vi "MI Sync with Triggering (MAIN) repeatability.vi"(10 "FGENs":refnum<k15>[](array[refnum])=["FGEN1", "FGEN2"] caption="Resource Name", 11 "Scopes":refnum<k15>[](array[refnum])=["SCOPE1", "SCOPE2"] caption="resource name") -> (2 "Waveform Graph":waveform(dbl)[](graph), 3 "relative trigger position (s)":dbl[](array[numeric]) format="%#.3p")   [LabVIEW 2024]
doc: "This VI is a one shot example of synchronising 2x arb with 2 and 1 channels with 2x scopes with 2 and 1 channel.\nThe frequency the arb are to produce is set on the front panel and all are identical amplitude and frequency with the phase set to a 120 degree difference.\nTriggering of the oscilloscope is based on channel 0 of the first specified scope module as the signal crosses zero.\nWIthout using TCLK, triggering happens by preparing the FGEN first and starting their output when the master SCOPE which is set to reference trigger on ch0 passes out it's ready for start event. The second scope uses the reference trigger event from the first scope to start."
uses:
  <instrlib>/niScope/Acquire/Fetch/niScope Multi Fetch WDT.vi
  <vilib>/measure/matone.llb/Extract Single Tone Information N Chan.vi
  <vilib>/measure/NI_MAPro.lvlib
  <vilib>/Analysis/NI_AALBase.lvlib
panel:
  out "Progress":dbl(slide) scale=0.0..100.0
  out "min relative trigger position":dbl
  out "max relative trigger position":dbl format="%#_6p"
  in  "Number of repeats":i32=1
  out "Histogram Graph Relative Trigger Positions":T1(graph)
  out "detected frequencies (Hz)":dbl[](array[numeric])
  out "detected phases (deg)":dbl[](array[numeric])
  # "Hardware Configuration"
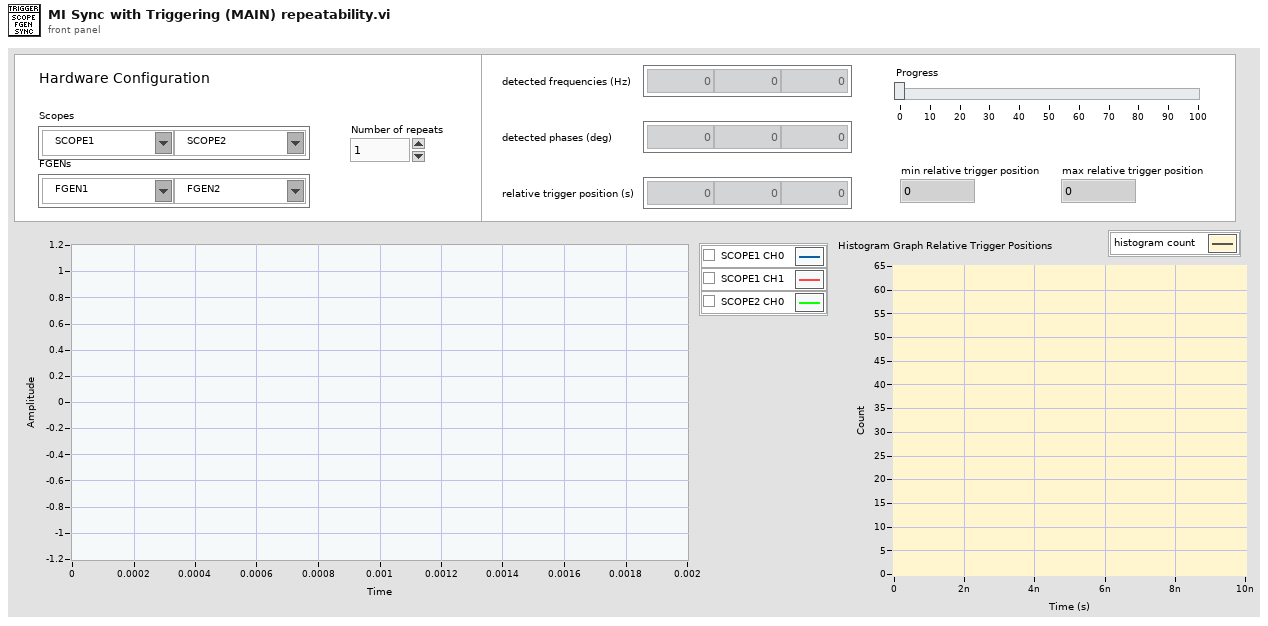
[diagram p1: front panel]
types:
  T1 = cluster{"X Values":dbl[], "Histogram: h(x)":i32[]}
  T2 = cluster{"actualSamples":i32, "absoluteInitialX":dbl, "relativeInitialX":dbl, "xIncrement":dbl, "offset":dbl, "gain":dbl, "reserved1":dbl, "reserved2":dbl}[]
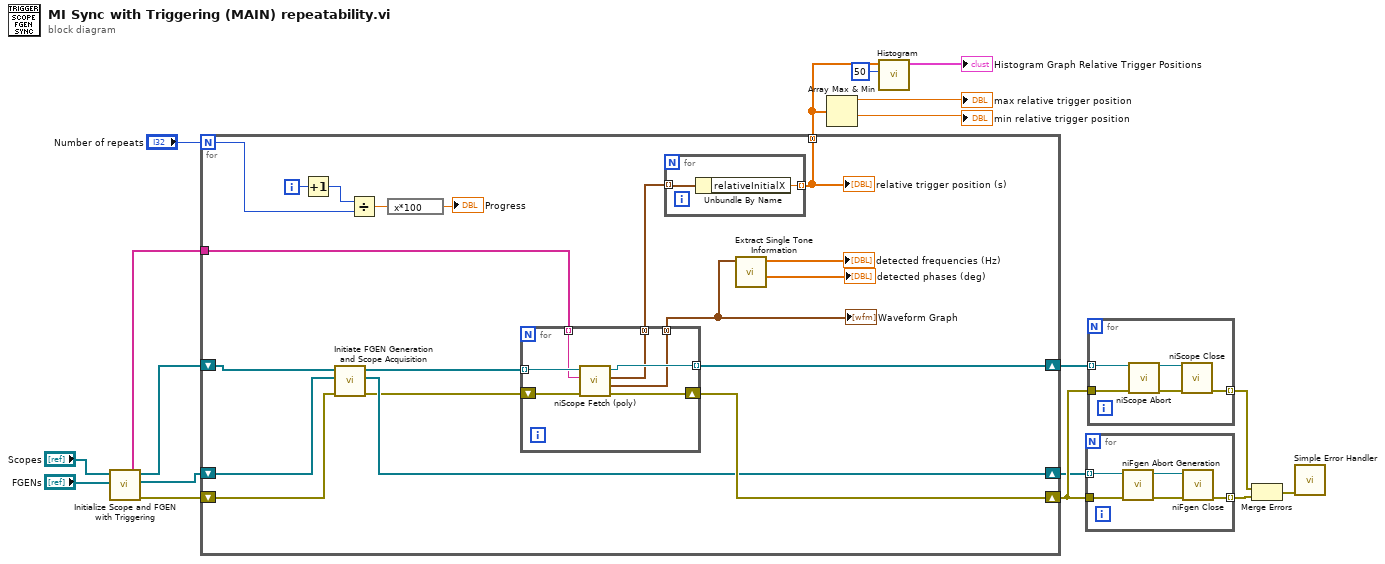
[diagram p0: block diagram]
diagram:
  n1 = call "Initialize Scope and FGEN with Triggering.vi"("FGEN Resources in"="FGENs", "Scope Resources in"="Scopes") -> ("error out"=w5:errorcluster, "FGEN Resources out"=w3:refnum<k15>[], "Scope Resources out"=w2:refnum<k15>[], "scope channels"=w1:string[])  [unwired: 6 in]
  n2 = for {
    N: "Number of repeats" -> [w28]
    tunnel: w1 -> [w36]
    tunnel: [w31] -> w4 mode=concatenating
    shift-right: [w22] -> w6
    shift-left: w3 -> [w23]
    shift-right: [w37] -> w17
    shift-left: w2 -> [w25]
    shift-right: [w35] -> w13
    shift-left: w5 -> [w20]
    i -> [w30]
    n3 = Increment(x=w30) -> (x+1=w29:i32)
    n4 = call "Initiate FGEN Generation and Scope Acquisition.vi"("error in (no error)"=w20, "FGEN Resources in"=w23, "Scope Resources in"=w25) -> ("error out"=w21:errorcluster, "FGEN Resources out"=w22:refnum<k15>[], "Scope Resources out"=w24:refnum<k15>[])  [unwired: 6 in]
    n5 = Divide(x=w29, y=w28) -> (x/y=w27:dbl)
    n6 = expression code="x*100"(w27) -> (→"Progress":dbl)
    n7 = for {
      tunnel: w24 -> [w44] mode=indexing
      tunnel: [w43] -> w37 mode=indexing
      tunnel: [w41] -> w19 mode=concatenating
      tunnel: w36 -> [w40] mode=indexing
      tunnel: [w39] -> w32 mode=concatenating
      shift-right: [w42] -> w35
      shift-left: w21 -> [w38]
      n8 = call-poly <instrlib>:"niScope Fetch (poly).vi"("error in"=w38, "channels"=w40, "instrument handle"=w44) -> ("error out"=w42:errorcluster, "wfm"=w41:waveform(dbl)[], "wfm info"=w39:T2, "instrument handle out"=w43:refnum<k15>)  [unwired: 5 in]
    }
    "Waveform Graph" <- w19
    n9 = for {
      tunnel: w32 -> [w46] mode=indexing
      tunnel: [w45] -> w31 mode=indexing
      n10 = Unbundle By Name(w46) -> ("relativeInitialX"=w45:dbl)
    }
    "relative trigger position (s)" <- w31
    n11 = call-poly <vilib>:"Extract Single Tone Information.vi"("time signals in"=w19) -> ("detected phases (deg)"=→"detected phases (deg)":dbl[], "detected frequencies"=→"detected frequencies (Hz)":dbl[])  [unwired: 5 in, 4 out]
  }
  n12 = Array Max & Min(array=w4) -> (max value=→"max relative trigger position":dbl, min value=→"min relative trigger position":dbl)  [unwired: 2 out]
  n13 = call <vilib>:"Histogram.vi"("intervals"=50, "X"=w4) -> ("Histogram Graph"=→"Histogram Graph Relative Trigger Positions":T1)  [unwired: 6 in, 3 out]
  n14 = for {
    tunnel: w6 -> [w51] mode=indexing
    tunnel: [w50] -> w16 mode=indexing
    tunnel: w13 -> [w49]
    n15 = call <instrlib>:"niFgen Abort Generation.vi"("error in (no error)"=w49, "Instrument Handle"=w51) -> ("error out"=w48:errorcluster, "Instrument Handle Out"=w47:refnum<k15>)  [unwired: 8 in]
    n16 = call <instrlib>:"niFgen Close.vi"("error in (no error)"=w48, "Instrument Handle"=w47) -> ("error out"=w50:errorcluster)  [unwired: 9 in]
  }
  n17 = for {
    tunnel: w17 -> [w56] mode=indexing
    tunnel: w13 -> [w55]
    tunnel: [w54] -> w15 mode=indexing
    n18 = call <instrlib>:"niScope Abort.vi"("instrument handle"=w56, "error in"=w55) -> ("instrument handle out"=w53:refnum<k15>, "error out"=w52:errorcluster)  [unwired: 12 in]
    n19 = call <instrlib>:"niScope Close.vi"("instrument handle"=w53, "error in"=w52) -> ("error out"=w54:errorcluster)  [unwired: 13 in]
  }
  n20 = Merge Errors(w15, w16) -> (w12:errorcluster)
  n21 = call <vilib>:"Simple Error Handler.vi"("error in (no error)"=w12) -> ()  [unwired: 4 in, 5 out]
